vi "Replace timestamp.vi"(10 "Array 2":waveform(dbl)[](array[waveform]), 11 "Array 1":waveform(dbl)[](array[waveform])) -> (3 "Array Out":waveform(dbl)[](array[waveform]))   [LabVIEW 2016, in "DSP_lockin.lvclass"]
uses:
  DSP_lockin.lvclass
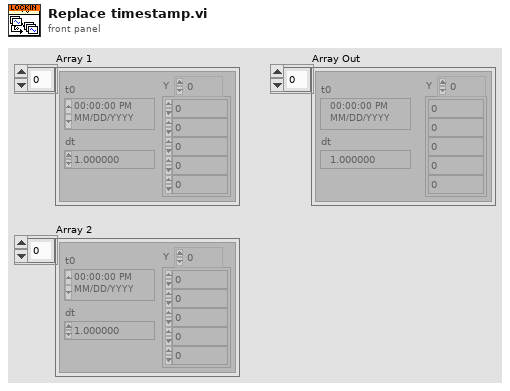
[diagram p1: front panel]
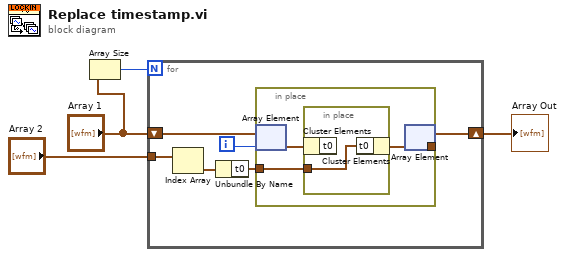
[diagram p0: block diagram]
diagram:
  n1 = Array Size(array="Array 1") -> (size(s)=w2:i32)
  n2 = for {
    N: w2 -> [_]
    tunnel: "Array 2" -> [w9]
    shift-right: [w5] -> w1
    shift-left: "Array 1" -> [w8]
    i -> [w6]
    n3 = Index Array(array=w9) -> (element=w10:waveform(dbl))  [unwired: 1 in]
    n4 = Unbundle By Name(w10) -> ("t0"=w7:timestamp)
    n5 = in-place {
      in-place-border: w7 -> [w12]
      in-place-border: [w11] -> _
      n6 = in-place-array #1(w8, w6) -> (w13:waveform(dbl))
      n7 = in-place {
        in-place-border: w12 -> [w14]
        n8 = in-place-cluster #2(w13) -> ()  [unwired: 1 out]
        n9 = in-place-cluster #2("t0"=w14) -> (w11:waveform(dbl))
      }
      n10 = in-place-array #1(w11) -> (w5:waveform(dbl)[])  [unwired: 1 out]
    }
  }
  "Array Out" <- w1
